vi "串口小助手.vi"() -> ()   [LabVIEW 2016]
uses:
  <vilib>/Instr/_visa.llb/VISA Configure Serial Port (Instr).vi
panel:
  in  "ID":string
  in  "间隔/ms":dbl=100.0
  in  "循环发送":bool
  in  "发送十六进制显示":bool
  in  "接收十六进制显示":bool
  in  "清除计数":bool
  in  "清除发送区":bool
  in  "清除接收区":bool
  in  "停止运行":bool
  in  "接收区自动清空":bool
  out "接收数目":u32
  out "接收总数":u32
  out "接收错误状态":bool
  out "发送总数":u32
  out "发送数目":u32
  out "发送错误状态":bool
  in  "发送":bool
  out "接收":string
  in  "发送":string
  out "VISA资源名称输出":refnum<visa-resource-name>
  out "status":bool
  in  "baud rate (9600)":u32(ring)=9600 caption="波特率" items=["9600"=9600, "19200"=19200, "115200"=115200, ""=0]
  in  "VISA resource name":refnum<visa-resource-name> caption="串口号"
  in  "关闭串口":bool
  in  "打开串口":bool
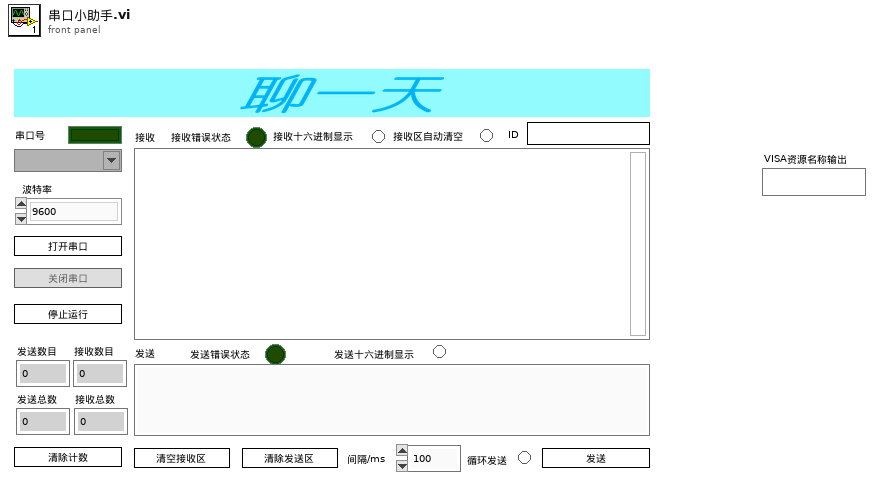
[diagram p1: front panel]
types:
  T1 = enum8{"Enabled", "Disabled", "Disabled and Grayed Out"}
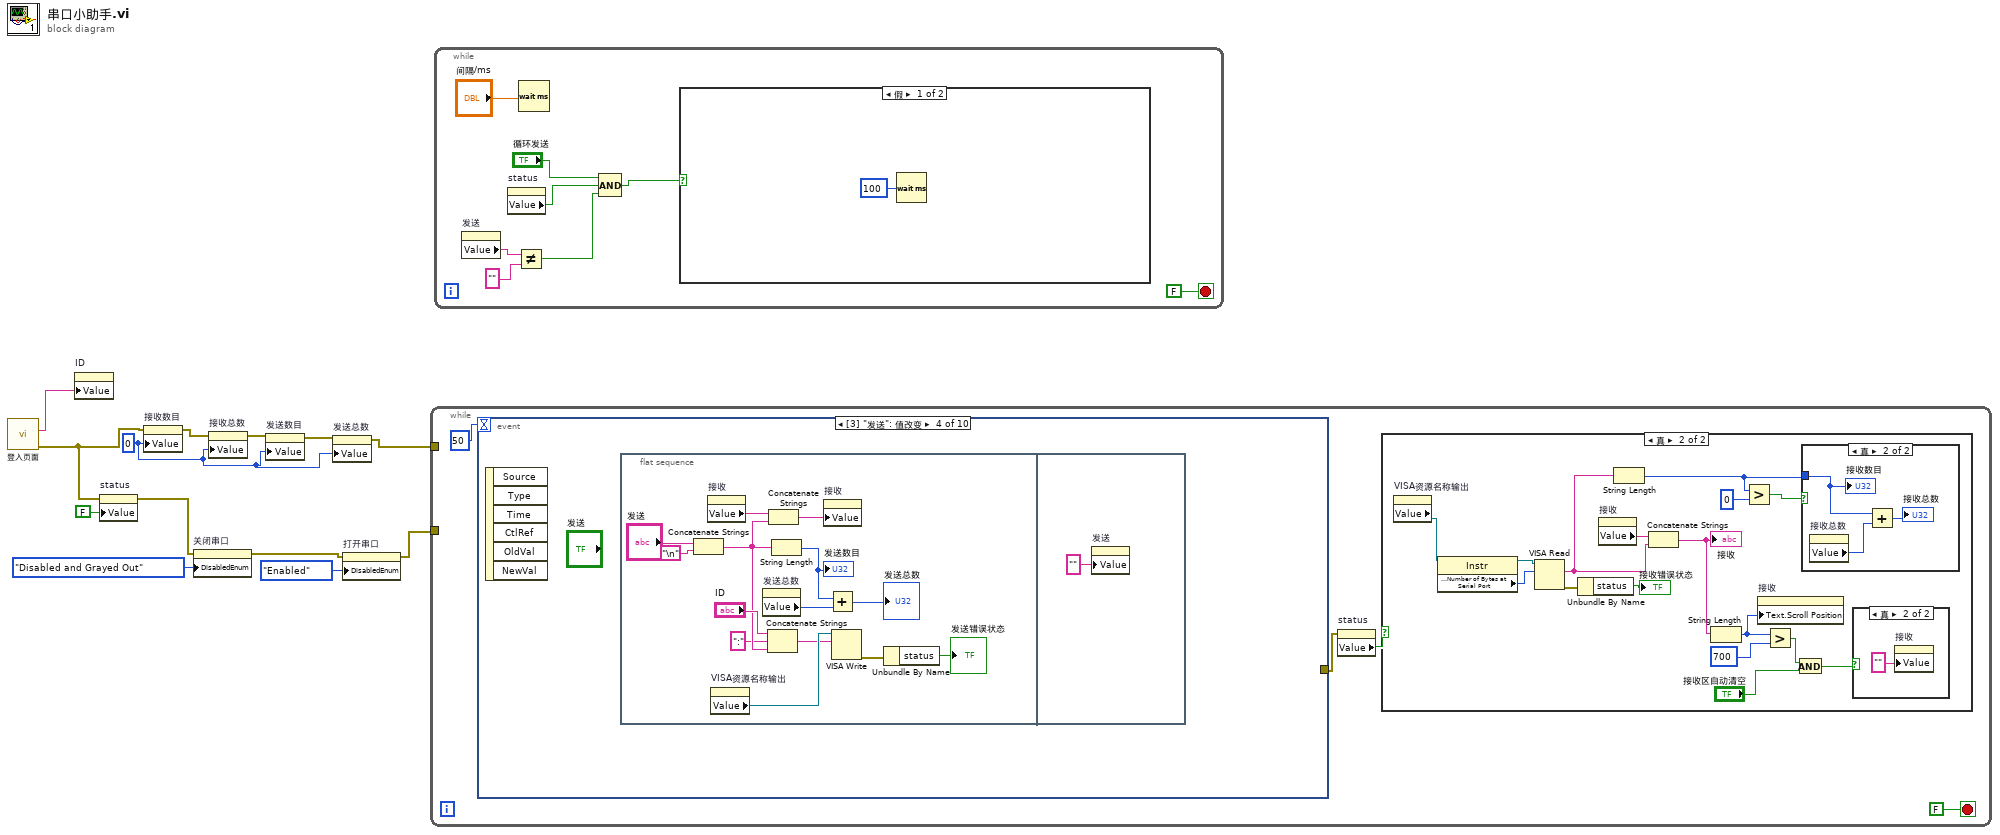
[diagram p0: block diagram]
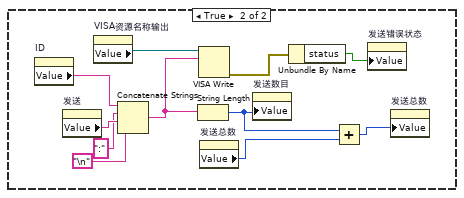
[diagram p2: hidden frame]
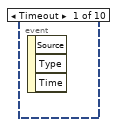
[diagram p6: hidden frame]
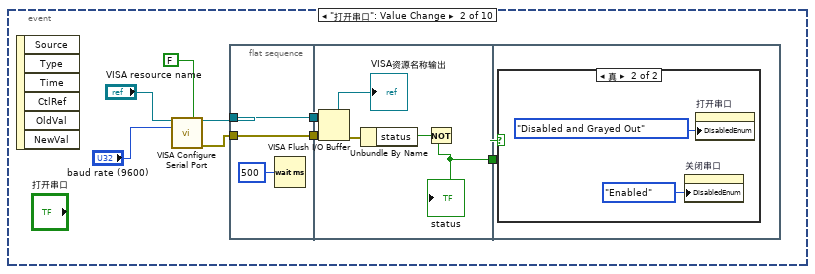
[diagram p7: hidden frame]
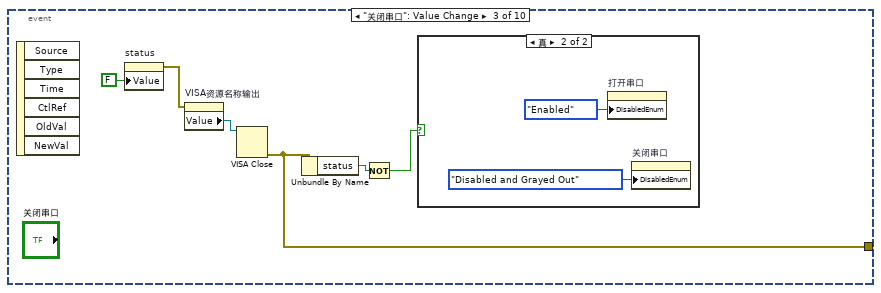
[diagram p9: hidden frame]
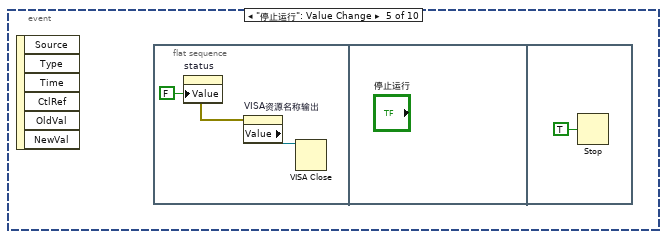
[diagram p11: hidden frame]
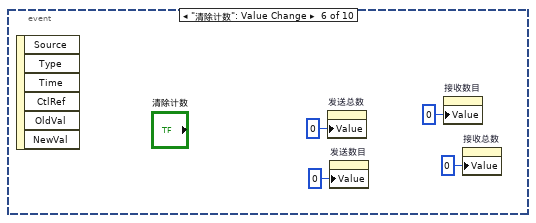
[diagram p12: hidden frame]
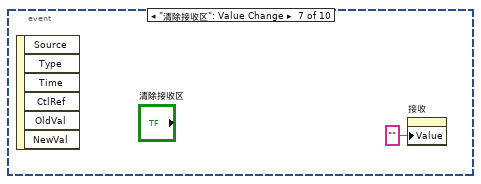
[diagram p13: hidden frame]
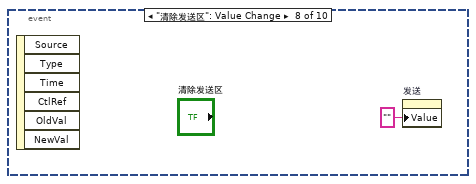
[diagram p14: hidden frame]
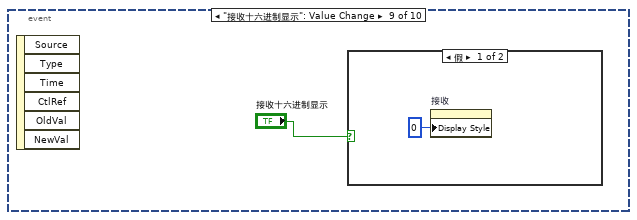
[diagram p15: hidden frame]
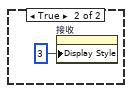
[diagram p16: hidden frame]
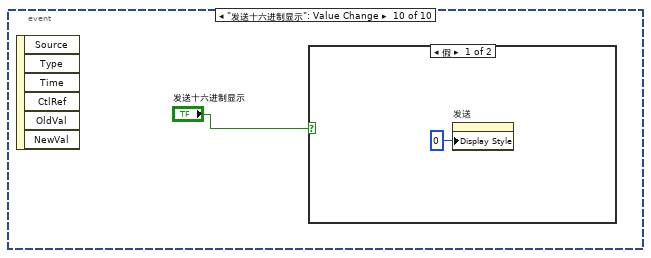
[diagram p17: hidden frame]
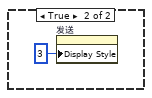
[diagram p18: hidden frame]
diagram:
  w3 = u32 0 ("接收数目")
  n1 = call "登入页面.vi"() -> ("登入人名字"=w1:string, "error out"=w2:errorcluster)  [unwired: 8 in, 1 out]
  n2 = property on="ID" class="Str"("Value"=w1) -> ()  [unwired: 2 in, 2 out]
  n3 = property on="status" class="Bool (严格)"(error in=w2, "Value"=FALSE ("status")) -> (error out=w9:errorcluster)  [unwired: 1 in, 1 out]
  n4 = property on="接收数目" class="DigNum (严格)"(error in=w2, "Value"=w3) -> (error out=w7:errorcluster)  [unwired: 1 in, 1 out]
  n5 = property on="关闭串口" class="Bool (严格)"(error in=w9, "DisabledEnum"=T1."Disabled and Grayed Out" ("禁用")) -> (error out=w11:errorcluster)  [unwired: 1 in, 1 out]
  n6 = property on="接收总数" class="DigNum (严格)"(error in=w7, "Value"=w3) -> (error out=w6:errorcluster)  [unwired: 1 in, 1 out]
  n7 = property on="发送数目" class="DigNum (严格)"(error in=w6, "Value"=w3) -> (error out=w5:errorcluster)  [unwired: 1 in, 1 out]
  n8 = property on="发送总数" class="DigNum (严格)"(error in=w5, "Value"=w3) -> (error out=w4:errorcluster)  [unwired: 1 in, 1 out]
  n9 = property on="打开串口" class="Bool (严格)"(error in=w11, "DisabledEnum"=T1."Enabled" ("禁用")) -> (error out=w10:errorcluster)  [unwired: 1 in, 1 out]
  n10 = while {
    tunnel: w10 -> [_]
    tunnel: w4 -> [_]
    stop <- FALSE stop-if-true
    n11 = event shown="[3] \"发送\": 值改变" {
      selector: _ -> [_ _ _ _ _ _ _ _ _ _]
      dyn-events: _ -> [_ _ _ _ _ _ _ _ _ _]
      timeout: 50 -> [_ _ _ _ _ _ _ _ _ _]
      tunnel: [_ _ w58 _ _ _ _ _ _ _] -> w14
      event Timeout {
        n12 = event-data() -> ()  [unwired: 1 in, 3 out]
      }
      event "打开串口": Value Change {
        n13 = event-data() -> ()  [unwired: 1 in, 6 out]
        n14 = call-poly "VISA Configure Serial Port"("VISA resource name"="VISA resource name", "Enable Termination\nChar (T)"=FALSE ("Enable Termination\nChar (T)"), "baud rate (9600)"="baud rate (9600)") -> ("VISA resource name out"=w42:refnum<visa-resource-name>, "error out"=w39:errorcluster)  [unwired: 11 in]
        n15 = flat-sequence {
          tunnel: w42 -> [w47]
          tunnel: [w47] -> w41
          tunnel: [w46] -> w40
          tunnel: w39 -> [w46]
          tunnel: w41 -> [w54]
          tunnel: w40 -> [w53]
          tunnel: [w49] -> w38
          tunnel: w38 -> [w55]
          frame #0 {
            n16 = Wait (ms)(milliseconds to wait=u32 500 ("等待时间（毫秒）")) -> ()  [unwired: 1 out]
          }
          frame #1 {
            n17 = VISA Flush I/O Buffer(VISA resource name=w54, error in (no error)=w53) -> (VISA resource name out=→"VISA资源名称输出":refnum<visa-resource-name>, error out=w52:errorcluster)  [unwired: 1 in]
            n18 = Unbundle By Name(w52) -> ("status"=w51:bool)
            n19 = Not(x=w51) -> (.not. x?=w49:bool)
            "status" <- w49
          }
          frame #2 {
            n20 = case shown="真" w55 {
              frame False {
              }
              frame True {
                n21 = property on="关闭串口" class="Bool (严格)"("DisabledEnum"=T1."Enabled" ("禁用")) -> ()  [unwired: 2 in, 2 out]
                n22 = property on="打开串口" class="Bool (严格)"("DisabledEnum"=T1."Disabled and Grayed Out" ("禁用")) -> ()  [unwired: 2 in, 2 out]
              }
            }
          }
        }
      }
      event "关闭串口": Value Change {
        n23 = event-data() -> ()  [unwired: 1 in, 6 out]
        n24 = property on="status" class="Bool (严格)"("Value"=FALSE ("status")) -> (error out=w59:errorcluster)  [unwired: 2 in, 1 out]
        n25 = property on="VISA资源名称输出" class="VISAName"(error in=w59) -> ("Value"=w63:refnum<visa-resource-name>)  [unwired: 1 in, 2 out]
        n26 = VISA Close(VISA resource name=w63) -> (error out=w58:errorcluster)  [unwired: 1 in]
        n27 = Unbundle By Name(w58) -> ("status"=w62:bool)
        n28 = Not(x=w62) -> (.not. x?=w61:bool)
        n29 = case shown="真" w61 {
          frame False {
          }
          frame True {
            n30 = property on="打开串口" class="Bool (严格)"("DisabledEnum"=T1."Enabled" ("禁用")) -> ()  [unwired: 2 in, 2 out]
            n31 = property on="关闭串口" class="Bool (严格)"("DisabledEnum"=T1."Disabled and Grayed Out" ("禁用")) -> ()  [unwired: 2 in, 2 out]
          }
        }
      }
      event "发送": Value Change {
        n32 = event-data() -> ()  [unwired: 1 in, 6 out]
        n33 = flat-sequence {
          frame #0 {
            n34 = Concatenate Strings("发送", "\n") -> (w67:string)
            n35 = property on="接收" class="Str"() -> ("Value"=w71:string)  [unwired: 2 in, 2 out]
            n36 = property on="VISA资源名称输出" class="VISAName"() -> ("Value"=w79:refnum<visa-resource-name>)  [unwired: 2 in, 2 out]
            n37 = property on="发送总数" class="DigNum (严格)"() -> ("Value"=w75:u32)  [unwired: 2 in, 2 out]
            n38 = Concatenate Strings("ID", ":", w67) -> (w69:string)
            n39 = Concatenate Strings(w71, w67) -> (w70:string)
            n40 = String Length(string=w67) -> (length=w76:i32)
            "发送数目" <- w76
            n41 = property on="接收" class="Str"("Value"=w70) -> ()  [unwired: 2 in, 2 out]
            n42 = Add(x=w76, y=w75) -> (x+y=→"发送总数":u32)
            n43 = VISA Write(VISA resource name=w79, write buffer=w69) -> (error out=w78:errorcluster)  [unwired: 1 in, 2 out]
            n44 = Unbundle By Name(w78) -> ("status"=→"发送错误状态":bool)
          }
          frame #1 {
            n45 = property on="发送" class="Str"("Value"="" ("发送内容")) -> ()  [unwired: 2 in, 2 out]
          }
        }
      }
      event "停止运行": Value Change {
        n46 = event-data() -> ()  [unwired: 1 in, 6 out]
        n47 = flat-sequence {
          frame #0 {
            n48 = property on="status" class="Bool (严格)"("Value"=FALSE ("status")) -> (error out=w81:errorcluster)  [unwired: 2 in, 1 out]
            n49 = property on="VISA资源名称输出" class="VISAName"(error in=w81) -> ("Value"=w83:refnum<visa-resource-name>)  [unwired: 1 in, 2 out]
            n50 = VISA Close(VISA resource name=w83) -> ()  [unwired: 1 in, 1 out]
          }
          frame #1 {
          }
          frame #2 {
            n51 = Stop(stop? (T)=TRUE ("停止？(T)")) -> ()
          }
        }
      }
      event "清除计数": Value Change {
        n52 = event-data() -> ()  [unwired: 1 in, 6 out]
        n53 = property on="发送总数" class="DigNum (严格)"("Value"=u32 0 ("发送总数")) -> ()  [unwired: 2 in, 2 out]
        n54 = property on="发送数目" class="DigNum (严格)"("Value"=u32 0 ("发送数目")) -> ()  [unwired: 2 in, 2 out]
        n55 = property on="接收数目" class="DigNum (严格)"("Value"=u32 0 ("接收数目")) -> ()  [unwired: 2 in, 2 out]
        n56 = property on="接收总数" class="DigNum (严格)"("Value"=u32 0 ("接收总数")) -> ()  [unwired: 2 in, 2 out]
      }
      event "清除接收区": Value Change {
        n57 = event-data() -> ()  [unwired: 1 in, 6 out]
        n58 = property on="接收" class="Str"("Value"="" ("接收内容")) -> ()  [unwired: 2 in, 2 out]
      }
      event "清除发送区": Value Change {
        n59 = event-data() -> ()  [unwired: 1 in, 6 out]
        n60 = property on="发送" class="Str"("Value"="" ("发送内容")) -> ()  [unwired: 2 in, 2 out]
      }
      event "接收十六进制显示": Value Change {
        n61 = event-data() -> ()  [unwired: 1 in, 6 out]
        n62 = case shown="假" "接收十六进制显示" {
          frame False {
            n63 = property on="接收" class="Str"("Display Style"=u32 0 ("显示样式")) -> ()  [unwired: 2 in, 2 out]
          }
          frame True {
            n64 = property on="接收" class="Str"("Display Style"=u32 3 ("显示样式")) -> ()  [unwired: 2 in, 2 out]
          }
        }
      }
      event "发送十六进制显示": Value Change {
        n65 = event-data() -> ()  [unwired: 1 in, 6 out]
        n66 = case shown="假" "发送十六进制显示" {
          frame False {
            n67 = property on="发送" class="Str"("Display Style"=u32 0 ("显示样式")) -> ()  [unwired: 2 in, 2 out]
          }
          frame True {
            n68 = property on="发送" class="Str"("Display Style"=u32 3 ("显示样式")) -> ()  [unwired: 2 in, 2 out]
          }
        }
      }
    }
    n69 = property on="status" class="Bool (严格)"(error in=w14) -> ("Value"=w15:bool)  [unwired: 1 in, 2 out]
    n70 = case shown="真" w15 {
      frame False {
      }
      frame True {
        n71 = property on="VISA资源名称输出" class="VISAName"() -> ("Value"=w31:refnum<visa-resource-name>)  [unwired: 2 in, 2 out]
        n72 = property class="Instr"(reference=w31) -> (reference out=w33:refnum<visa-resource-name>, "Serial Settings:Number of Bytes at Serial Port"=w32:u32)  [unwired: 1 in, 1 out]
        n73 = VISA Read(VISA resource name=w33, byte count=w32) -> (read buffer=w27:string, error out=w28:errorcluster)  [unwired: 1 in, 2 out]
        n74 = Unbundle By Name(w28) -> ("status"=→"接收错误状态":bool)
        n75 = property on="接收" class="Str"() -> ("Value"=w30:string)  [unwired: 2 in, 2 out]
        n76 = String Length(string=w27) -> (length=w20:i32)
        n77 = Concatenate Strings(w30, w27) -> (w26:string)
        "接收" <- w26
        n78 = String Length(string=w26) -> (length=w18:i32)
        n79 = Greater?(x=w20, y=0) -> (0:w21:bool)
        n80 = property on="接收" class="Str"("Text.Scroll Position"=w18) -> ()  [unwired: 2 in, 2 out]
        n81 = Greater?(x=w18, y=700) -> (0:w24:bool)
        n82 = And(x=w24, y="接收区自动清空") -> (x .and. y?=w22:bool)
        n83 = case shown="真" w21 {
          tunnel: w20 -> [_ w34]
          frame False {
          }
          frame True {
            n84 = property on="接收总数" class="DigNum (严格)"() -> ("Value"=w35:u32)  [unwired: 2 in, 2 out]
            n85 = Add(x=w34, y=w35) -> (x+y=→"接收总数":u32)
            "接收数目" <- w34
          }
        }
        n86 = case shown="真" w22 {
          frame False {
          }
          frame True {
            n87 = property on="接收" class="Str"("Value"="" ("接收内容")) -> ()  [unwired: 2 in, 2 out]
          }
        }
      }
    }
  }
  n88 = while {
    stop <- FALSE stop-if-true
    n89 = property on="发送" class="Str"() -> ("Value"=w102:string)  [unwired: 2 in, 2 out]
    n90 = property on="status" class="Bool (严格)"() -> ("Value"=w99:bool)  [unwired: 2 in, 2 out]
    n91 = Not Equal?(x=w102, y="") -> (x != y?=w98:bool)
    n92 = Wait (ms)(milliseconds to wait="间隔/ms") -> ()  [unwired: 1 out]
    n93 = Compound Arithmetic op=AND ("复合运算")("循环发送", w99, w98) -> (w97:bool)
    n94 = case shown="假" w97 {
      frame False {
        n95 = Wait (ms)(milliseconds to wait=u32 100 ("等待时间（毫秒）")) -> ()  [unwired: 1 out]
      }
      frame True {
        n96 = property on="ID" class="Str"() -> ("Value"=w108:string)  [unwired: 2 in, 2 out]
        n97 = property on="发送" class="Str"() -> ("Value"=w110:string)  [unwired: 2 in, 2 out]
        n98 = property on="VISA资源名称输出" class="VISAName"() -> ("Value"=w115:refnum<visa-resource-name>)  [unwired: 2 in, 2 out]
        n99 = Concatenate Strings(w108, ":" ("字符串"), w110, "\n") -> (w107:string)
        n100 = String Length(string=w107) -> (length=w112:i32)
        n101 = VISA Write(VISA resource name=w115, write buffer=w107) -> (error out=w116:errorcluster)  [unwired: 1 in, 2 out]
        n102 = property on="发送总数" class="DigNum (严格)"() -> ("Value"=w113:u32)  [unwired: 2 in, 2 out]
        n103 = property on="发送数目" class="DigNum (严格)"("Value"=w112) -> ()  [unwired: 2 in, 2 out]
        n104 = Unbundle By Name(w116) -> ("status"=w114:bool)
        n105 = Add(x=w112, y=w113) -> (x+y=w111:u32)
        n106 = property on="发送错误状态" class="Bool (严格)"("Value"=w114) -> ()  [unwired: 2 in, 2 out]
        n107 = property on="发送总数" class="DigNum (严格)"("Value"=w111) -> ()  [unwired: 2 in, 2 out]
      }
    }
  }
